vi "Pause.vi"(8 "error in (no error)":errorcluster, 11 "FLOM Settings in":T1={"VISA resource name"="", "Simulated?"=FALSE, "Pump Number"=1.0} {"Pump Number" min=1.0 max=20.0 step=1.0}) -> (0 "error out":errorcluster, 1 "Connection Error":bool, 3 "FLOM Settings out":T1={"VISA resource name"="", "Simulated?"=FALSE, "Pump Number"=1.0} {"Pump Number" min=1.0 max=20.0 step=1.0})   [LabVIEW 2018, in "FLOM Pump.lvlib"]
uses:
  FLOM Pump.lvlib
  Settings Cluster.ctl
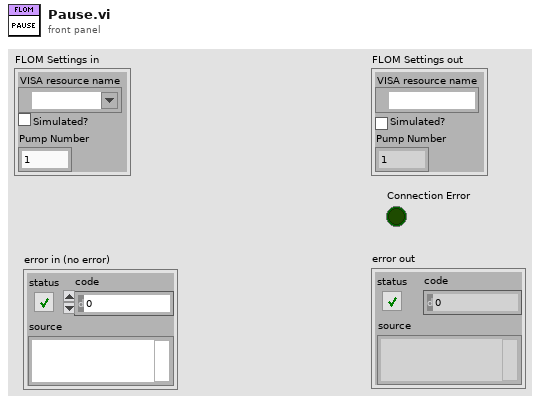
[diagram p1: front panel]
types:
  T1 = typedef "FLOM Pump.lvlib/Settings Cluster.ctl" = cluster{"VISA resource name":refnum<visa-resource-name>, "Simulated?":bool, "Pump Number":dbl}
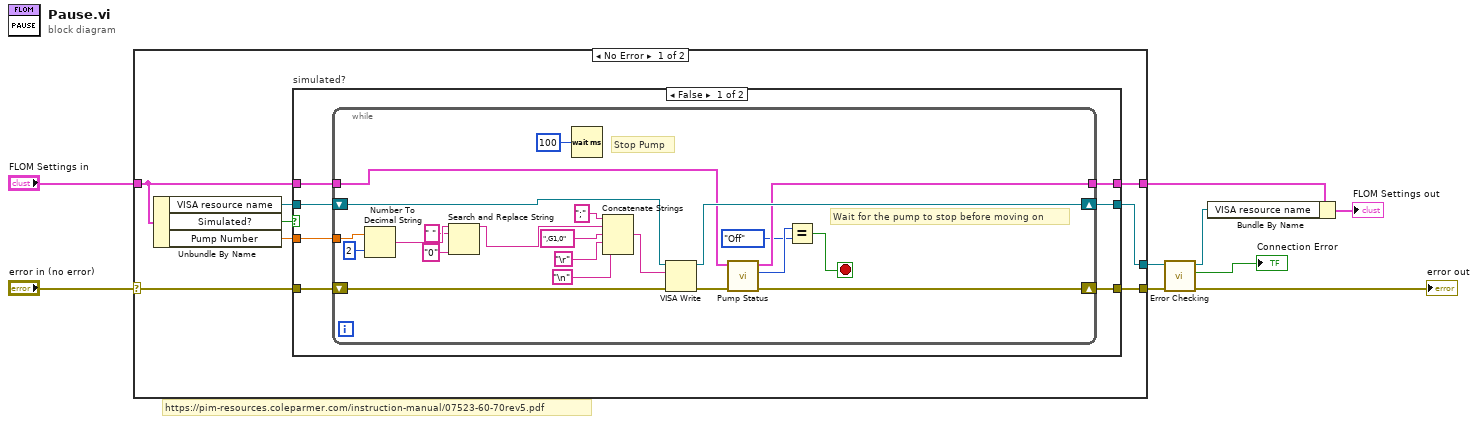
[diagram p0: block diagram]
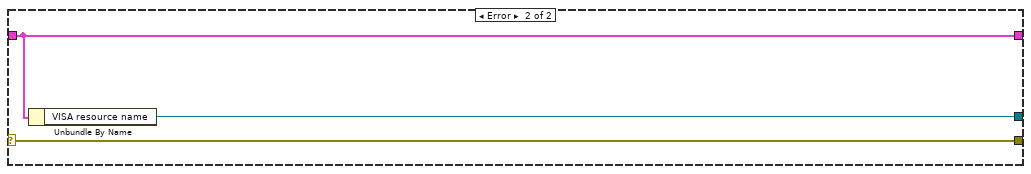
[diagram p3: hidden frame]
diagram:
  # "https://pim-resources.coleparmer.com/instruction-manual/07523-60-70rev5.pdf"
  n1 = case shown="No Error" "error in (no error)" {
    selector: "error in (no error)" -> [w15 w52]
    tunnel: [w11 w51] -> w9
    tunnel: "FLOM Settings in" -> [w12 w51]
    tunnel: [w14 w50] -> w6
    tunnel: [w13 w52] -> w7
    frame No Error {
      n2 = Unbundle By Name(w12) -> ("VISA resource name"=w17:refnum<visa-resource-name>, "Simulated?"=w16:bool, "Pump Number"=w10:dbl)
      n3 = case "simulated?" shown="False" w16 {
        tunnel: [w22 w49] -> w14
        tunnel: w17 -> [w24 w49]
        tunnel: w15 -> [w23 w48]
        tunnel: [w21 w48] -> w13
        tunnel: w12 -> [w20 w47]
        tunnel: [w19 w47] -> w11
        tunnel: w10 -> [w18 _]
        frame False {
          n4 = while {
            shift-right: [w44] -> w22
            shift-left: w24 -> [w46]
            shift-right: [w39] -> w21
            shift-left: w23 -> [w45]
            tunnel: w20 -> [w42]
            tunnel: [w41] -> w19
            tunnel: w18 -> [w25]
            stop <- w33 stop-if-true
            # "Wait for the pump to stop before moving on"
            # "Stop Pump"
            n5 = Number To Decimal String(number=w25, width (-)=i16 2) -> (decimal integer string=w29:string)
            n6 = Search and Replace String(input string=w29, search string=" ", replace string="0" ("replace string (\"\")")) -> (result string=w26:string)  [unwired: 5 in, 3 out]
            n7 = Wait (ms)(milliseconds to wait=u32 100) -> ()  [unwired: 1 out]
            n8 = Concatenate Strings(";" ("string"), w26, ",G1,0" ("string"), "\r", "\n") -> (w35:string)
            n9 = VISA Write(VISA resource name=w46, write buffer=w35, error in (no error)=w45) -> (VISA resource name out=w44:refnum<visa-resource-name>, error out=w40:errorcluster)  [unwired: 1 out]
            n10 = call "Pump Status.vi"("error in (no error)"=w40, "FLOM Settings In"=w42) -> ("error out"=w39:errorcluster, "Pump On?"=w34:enum16{"Off", "On", "Not Initialized"}, "FLOM Settings Out"=w41:T1)  [unwired: 4 in, 3 out]
            n11 = Equal?(x=w34, y=enum16{"Off", "On", "Not Initialized"}."Off") -> (x = y?=w33:bool)
          }
        }
        frame True {
        }
      }
    }
    frame Error {
      n12 = Unbundle By Name(w51) -> ("VISA resource name"=w50:refnum<visa-resource-name>)
    }
  }
  n13 = call "Error Checking.vi"("error in (no error)"=w7, "VISA resource name"=w6) -> ("error out"=→"error out":errorcluster, "Connection Error"=→"Connection Error":bool, "VISA resource name"=w8:refnum<visa-resource-name>)  [unwired: 7 in]
  n14 = Bundle By Name(cluster=w9, "VISA resource name"=w8) -> (→"FLOM Settings out":T1)
